vi "RT Driver VI.vi"(6 "Device Clock":string, 9 "Device Inputs FIFO":refnum<k33>, 10 "Device Outputs FIFO":refnum<k33>, 11 "Device Reference":T1 format="%.0x") -> ()   [LabVIEW 2020, in "Regatron G5 Custom Device Engine.lvlib"]
uses:
  Regatron G5 Custom Device Engine.lvlib
  <vilib>/NI VeriStand/Custom Device API/Custom Device Item Ref.ctl
  <vilib>/NI VeriStand/Custom Device API/Custom Device Channel Type.ctl
  <vilib>/Platform/TimedLoop/XDataNode/timing_clust.ctl
  <vilib>/Platform/TimedLoop/XDataNode/nitl_modes.ctl
  <vilib>/Platform/TimedLoop/XDataNode/wakeup.ctl
  G5 LabVIEW REST API/Regatron.G5.Rest Handle.llb/G5.Rest Status.ctl
  G5 LabVIEW REST API/Regatron.G5.Rest System.llb/G5.Rest System Output References Datasource.ctl
  G5 LabVIEW REST API/Regatron.G5.Rest System.llb/G5.Rest System Output Limits Datasource.ctl
  G5 LabVIEW REST API/Regatron.G5.Rest System.llb/G5.Rest System Output Limits.ctl
  G5 LabVIEW REST API/Regatron.G5.Rest System.llb/G5.Rest System Output References.ctl
  G5 LabVIEW REST API/Regatron.G5.Rest System.llb/G5.Rest System Clear Inicidents.ctl
  <userlib>/_OpenG.lib/array/array.llb/Search 1D Array (Boolean)__ogtk.vi
  <vilib>/platform/TimedLoop/XDataNode/XDataNode.xnode
  <vilib>/NI VeriStand/Custom Device API/Custom Device API.lvlib
  <vilib>/NI VeriStand/Custom Device Tools/Custom Device Utility Library/Custom Device Utility Library.lvlib
  <vilib>/Platform/TimedLoop/XDataNode/XDNodeRunTimeDep.lvlib
  G5 LabVIEW REST API/Regatron.G5.Rest.lvlib
panel:
  in  "Initialization Status Notifier":refnum<notifier>
  in  "Status Notifier":refnum<notifier>
  # "Custom Device Template\nv1.0"
  # "Use this template as a starting point for creating a custom device code module. The input controls shown here are specially named controls that the system will use to provide the device loop with data. The controls are not required for the device loop to run. For instance, if the device doesn't produce any output data, then you don't need the Device Outputs FIFO control. If you do use these controls, however, they need to have these exact names to be functional."
  # "The optional status notifier element is used to notify the RT engine of the last state of the custom device, and to indicate the device has completed execution. If this control is not used, a default No Error value is returned to the system when the device finishes execution.\n\nNote: This error state is not checked until the system shuts down. Use an output status channel to send more immediate status values to the system."
  # "This optional input can be used to send the VeriStand Engine the final status of the custom device initalization process. If this control exists on the custom device front panel, the VeriStand Engine will wait for a status update before starting up. If the custom device reports an error, that will abort the execution of the current configuration in the VeriStand Engine.\n\nThis control can be deleted if the custom device does not need to send the initialization status update."
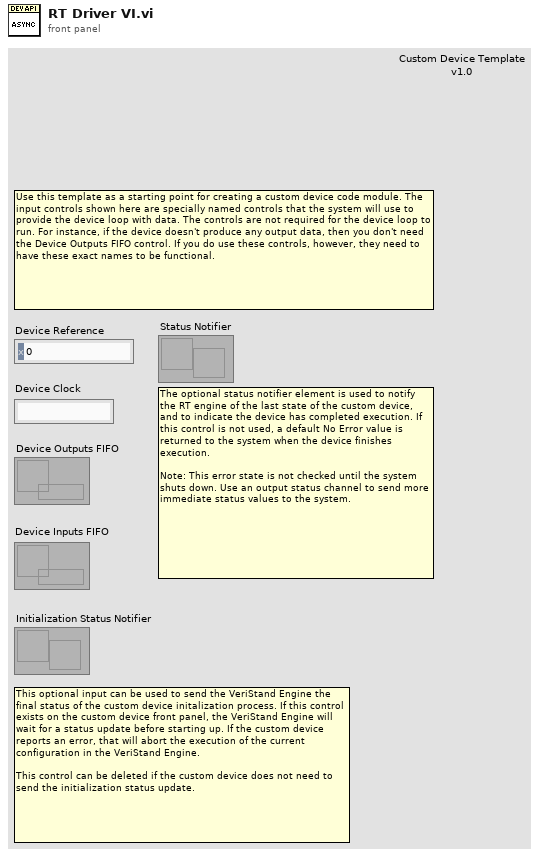
[diagram p1: front panel]
types:
  T1 = typedef "Custom Device API.lvlib/Custom Device Item Ref.ctl" = u64
  T2 = typedef "Custom Device API.lvlib/Custom Device Channel Type.ctl" = enum16{"Input", "Output"}
  T3 = typedef "XDNodeRunTimeDep.lvlib/nitl_modes.ctl" = enum32{"No Change", "Process missed periods, maintain original phase", "Discard missed periods, maintain original phase", "Process missed periods, ignore original phase", "Discard missed periods, ignore original phase"}
  T4 = typedef "XDNodeRunTimeDep.lvlib/timing_clust.ctl" = cluster{"Expected End [f-1]":u64, "Actual End [f-1]":u64, "Finished Late? [f-1]":bool, "Expected End [i-1]":u64, "Actual End [i-1]":u64, "Finished Late? [i-1]":bool, "Expected Start [i]":u64, "Actual Start [i]":u64, "Expected Start [f]":u64, "Actual Start [f]":u64, "Source Name":string, "Structure Name":string, "Period":i64, "Deadline":i64, "Offset":i64, "Start":i64, "Priority":i32, "Timeout":i32, "Mode":T3, "Wakeup Reason":T5, "Error":errorcluster, "Source Type":string, "Secondary Source Type":string, "Global End Time":u64, "Global Start Time":u64, "Frame Duration":u64, "Iteration Duration":u64, "Assigned CPU":i32, "I/O Scan Engine Mode":u32}
  T5 = typedef "XDNodeRunTimeDep.lvlib/wakeup.ctl" = enum32{"Normal", "Aborted", "Asynchronous wakeup", "Timing source error", "Timed loop error", "Timeout"}
  T6 = typedef "Regatron G5 Custom Device Shared.lvlib/Regatron.G5.Rest.lvlib/G5.Rest Status.ctl" = enum16{"Read", "Write"}
  T7 = typedef "Regatron G5 Custom Device Shared.lvlib/Regatron.G5.Rest.lvlib/G5.Rest System Output Limits.ctl" = cluster{"Voltage Upper Limit V":sgl, "Voltage Lower Limit V":sgl, "Current Upper Limit A":sgl, "Current Lower Limit A":sgl, "Power Upper Limit W":sgl, "Power Lower Limit W":sgl}
  T8 = typedef "Regatron G5 Custom Device Shared.lvlib/Regatron.G5.Rest.lvlib/G5.Rest System Output References.ctl" = cluster{"Voltage V":sgl, "Current A":sgl, "Power W":sgl, "Load R Ohm":sgl}
  T9 = typedef "Regatron G5 Custom Device Shared.lvlib/Regatron.G5.Rest.lvlib/G5.Rest System Clear Inicidents.ctl" = enum16{"Clear Errors and Warnings", "Clear Warnings", "Clear Errors"}
  T10 = typedef "Custom Device API.lvlib/Custom Device Timed Loop Priority.ctl" = enum32{"Low", "Medium", "High"}
  T11 = typedef "Regatron G5 Custom Device Shared.lvlib/Regatron.G5.Rest.lvlib/G5.Rest System Output References Datasource.ctl" = enum16{"Voltage", "Current", "Power", "Load Resistance", "ALL"}[]
  T12 = typedef "Regatron G5 Custom Device Shared.lvlib/Regatron.G5.Rest.lvlib/G5.Rest System Output Limits Datasource.ctl" = enum16{"Voltage Upper Limit", "Voltage Lower Limit", "Current Upper Limit", "Current Lower Limit", "Power Upper Limit", "Power Lower Limit", "ALL"}[]
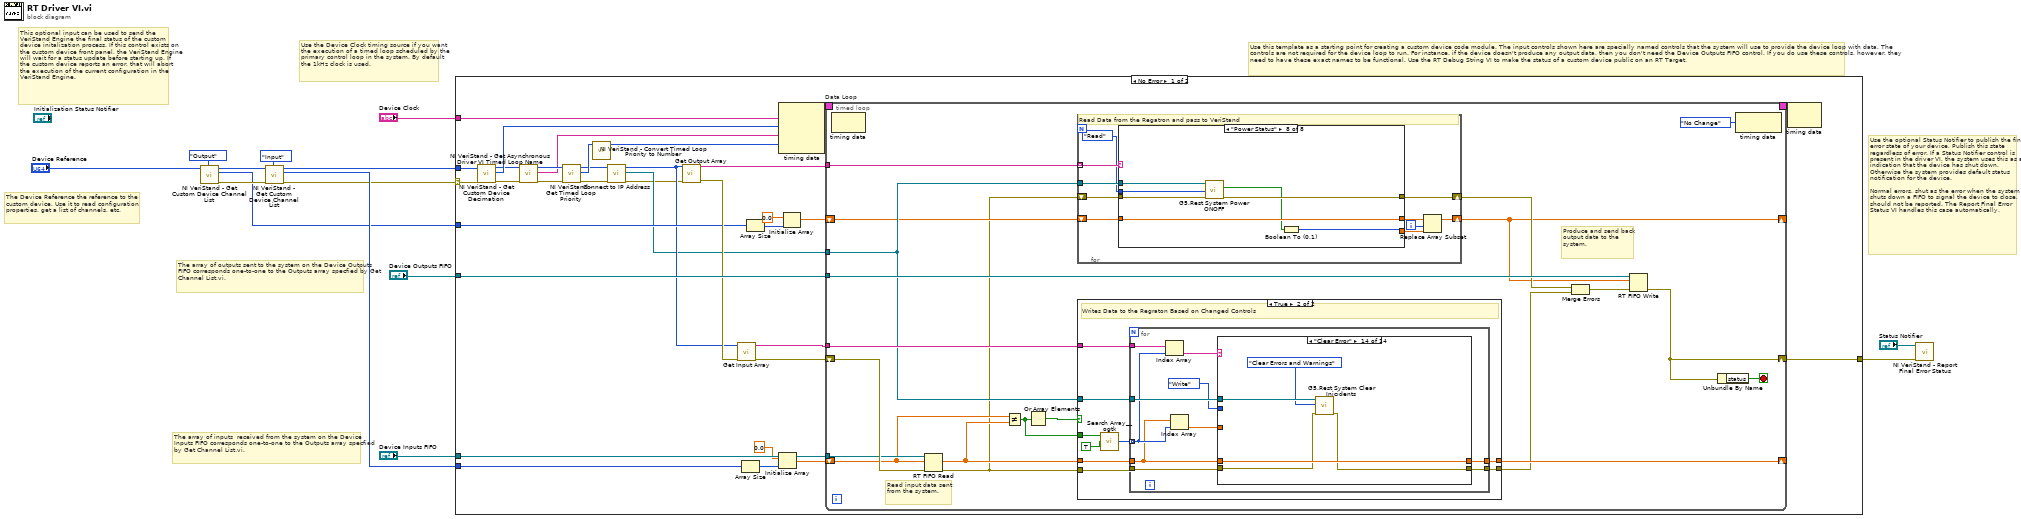
[diagram p0: block diagram]
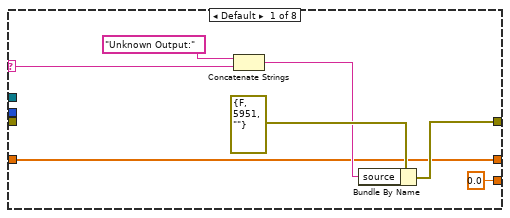
[diagram p2: hidden frame]
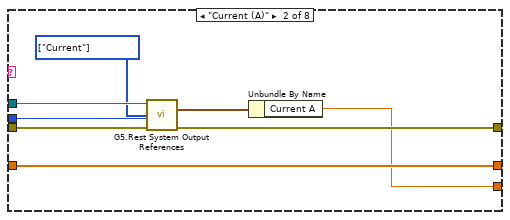
[diagram p3: hidden frame]
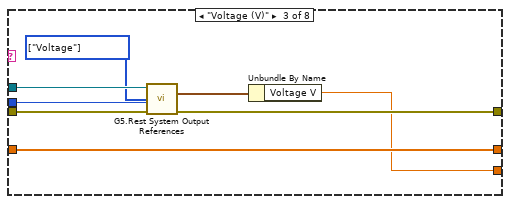
[diagram p4: hidden frame]
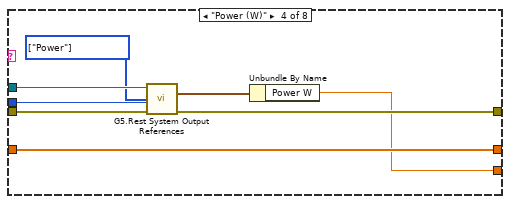
[diagram p5: hidden frame]
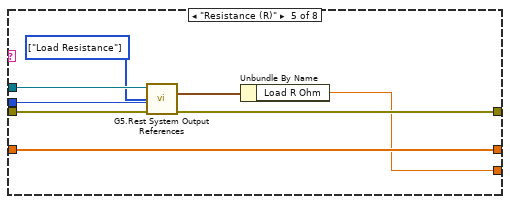
[diagram p6: hidden frame]
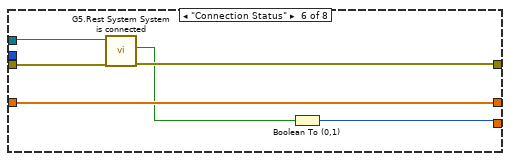
[diagram p7: hidden frame]
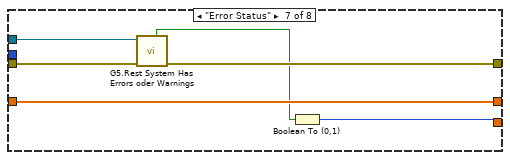
[diagram p8: hidden frame]
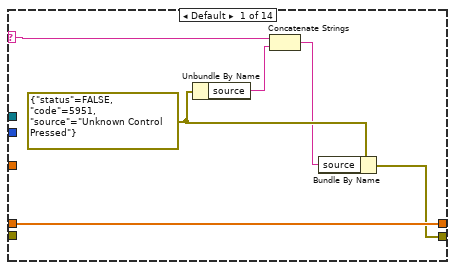
[diagram p10: hidden frame]
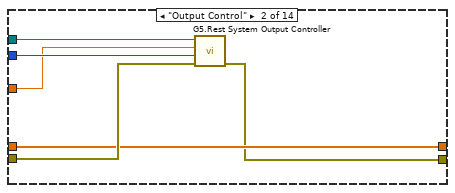
[diagram p11: hidden frame]
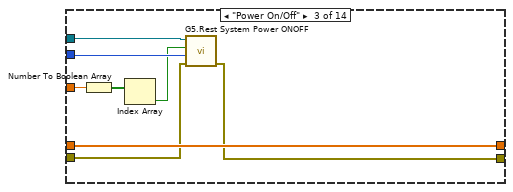
[diagram p12: hidden frame]
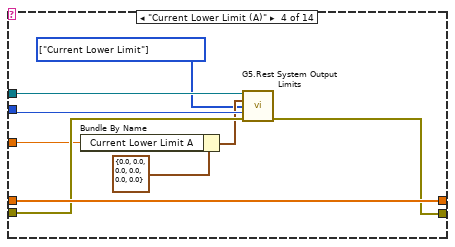
[diagram p13: hidden frame]
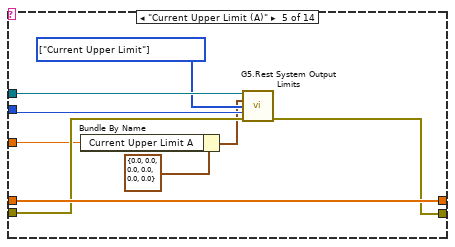
[diagram p14: hidden frame]
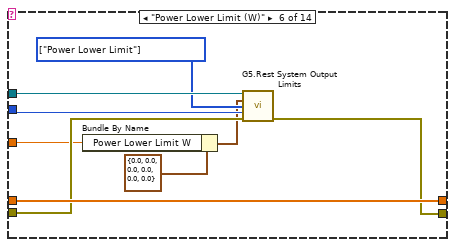
[diagram p15: hidden frame]
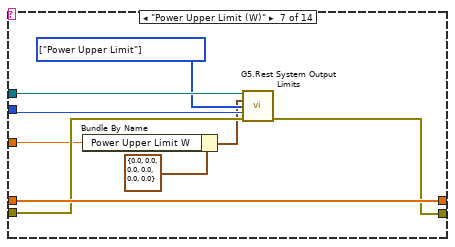
[diagram p16: hidden frame]
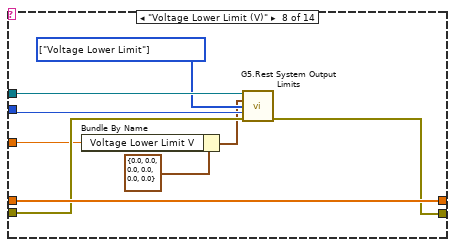
[diagram p17: hidden frame]
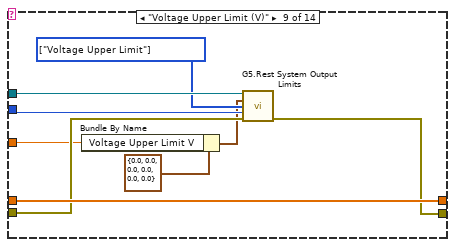
[diagram p18: hidden frame]
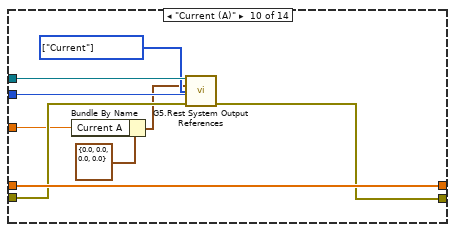
[diagram p19: hidden frame]
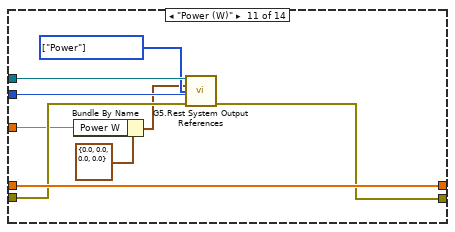
[diagram p20: hidden frame]
diagram:
  # "This optional input can be used to send the VeriStand Engine the final status of the custom device initalization process. If this control exists on the custom device front panel, the VeriStand Engine will wait for a status update before starting up. If the custom device reports an error, that will abort the execution of the current configuration in the VeriStand Engine."
  # "The array of inputs  received from the system on the Device Inputs FIFO corresponds one-to-one to the Outputs array specfied by Get Channel List.vi."
  # "Use the optional Status Notifier to publish the final error state of your device. Publish this state regardless of error. If a Status Notifier control is present in the driver VI, the system uses this as an indication that the device has shut down. Otherwise the system provides default status notification for the device.\n\nNormal errors, shut as the error when the system shuts down a FIFO to signal the device to close, should not be reported. The Report Final Error Status VI handles this case automatically."
  # "The array of outputs sent to the system on the Device Outputs FIFO corresponds one-to-one to the Outputs array specfied by Get Channel List.vi."
  # "The Device Reference the reference to the custom device. Use it to read configuration properties, get a list of channels, etc."
  # "Use the Device Clock timing source if you want the execution of a timed loop scheduled by the primary control loop in the system. By default the 1kHz clock is used."
  # "Use this template as a starting point for creating a custom device code module. The input controls shown here are specially named controls that the system will use to provide the device loop with data. The controls are not required for the device loop to run. For instance, if the device doesn't produce any output data, then you don't need the Device Outputs FIFO control. If you do use these controls, however, they need to have these exact names to be functional. Use the RT Debug String VI to make the status of a custom device public on an RT Target."
  n1 = call <vilib>:"NI VeriStand - Get Custom Device Channel List.vi"("Channel Type"=Custom_Device_Channel_Type."Output", "Device Ref in"="Device Reference") -> ("error out"=w11:errorcluster, "Specified Channel Ref List"=w2:T1[], "Device Ref out"=w5:T1)  [unwired: 1 in, 6 out]
  n2 = call <vilib>:"NI VeriStand - Get Custom Device Channel List.vi"("Channel Type"=Custom_Device_Channel_Type."Input", "error in (no error)"=w11, "Device Ref in"=w5) -> ("error out"=w3:errorcluster, "Specified Channel Ref List"=w9:T1[], "Device Ref out"=w4:T1)  [unwired: 6 out]
  n3 = case shown="No Error" w3 {
    selector: w3 -> [w31 w283]
    tunnel: "Device Outputs FIFO" -> [w47 _]
    tunnel: "Device Inputs FIFO" -> [w46 _]
    tunnel: w9 -> [w38 _]
    tunnel: [w39 w283] -> w6
    tunnel: w4 -> [w32 _]
    tunnel: w2 -> [w19 _]
    tunnel: "Device Clock" -> [w16 _]
    frame No Error {
      n4 = call <vilib>:"NI VeriStand - Get Custom Device Decimation.vi"("error in (no error)"=w31, "Device Ref in"=w32) -> ("error out"=w27:errorcluster, "Decimation"=w30:i32, "Device Ref out"=w28:T1)  [unwired: 7 in]
      n5 = call <vilib>:"NI VeriStand - Get Asynchronous Driver VI Timed Loop Name.vi"("error in (no error)"=w27, "Device Ref in"=w28) -> ("error out"=w26:errorcluster, "Device Timed Loop Name"=w24:string, "Device Ref out"=w25:T1)  [unwired: 7 in]
      n6 = call <vilib>:"NI VeriStand - Get Timed Loop Priority.vi"("error in (no error)"=w26, "Device Ref in"=w25) -> ("error out"=w20:errorcluster, "Priority"=w23:T10, "Device Ref out"=w21:T1)  [unwired: 7 in]
      n7 = call <vilib>:"NI VeriStand - Convert Timed Loop Priority to Number.vi"("Priority"=w23) -> ("Numeric Priority"=w22:i32)  [unwired: 10 in]
      n8 = call "Connect to IP Address.vi"("error in (no error)"=w20, "Device Ref in"=w21) -> ("error out"=w15:errorcluster, "REST Client out"=w17:refnum<class "REST Client.lvclass">, "Item Ref out"=w18:T1)  [unwired: 7 in]
      n9 = call "Get Output Array.vi"("error in"=w15, "Device Ref in"=w18) -> ("error out"=w29:errorcluster, "Array"=w35:string[])  [unwired: 8 in]
      n10 = call "Get Input Array.vi"("error in"=w29, "Device Ref in"=w18) -> ("error out"=w36:errorcluster, "Array"=w37:string[])  [unwired: 8 in]
      n11 = Array Size(array=w38) -> (size(s)=w40:i32)
      n12 = Array Size(array=w19) -> (size(s)=w41:i32)
      n13 = node-c288(w16, w30, w24, w22) -> (w34:T4)
      n14 = Initialize Array(0.0 ("element"), w40) -> (w42:dbl[])
      n15 = Initialize Array(0.0 ("element"), w41) -> (w43:dbl[])
      n16 = timed-loop "Data Loop" {
        shift-right: [w66] -> _
        shift-left: w42 -> [w62]
        shift-right: [w63] -> w39
        shift-left: w36 -> [w67]
        shift-right: [w50] -> _
        shift-left: w43 -> [w52]
        tunnel: w47 -> [w65]
        tunnel: w46 -> [w64]
        tunnel: w17 -> [w55]
        tunnel: w37 -> [w61]
        tunnel: w35 -> [w56]
        timing: w34 -> [_]
        timing-out: [_] -> w33
        stop <- w49 stop-if-true
        # "Produce and send back output data to the system."
        # "Read input data sent from the system."
        n17 = node-c288() -> ()  [unwired: 1 in, 1 out]
        n18 = RT FIFO Read(0:w64, 1:w62, 3:w67) -> (9:w58:dbl[], 11:w51:errorcluster)  [unwired: 4 out]
        n19 = Not Equal?(x=w62, y=w58) -> (x != y?=w60:bool[])
        n20 = Or Array Elements(Boolean array=w60) -> (logical OR=w57:bool)
        n21 = for {
          tunnel: w56 -> [w81] mode=indexing
          tunnel: w55 -> [w80]
          shift-right: [w79] -> w53
          shift-left: w51 -> [w77]
          shift-right: [w73] -> w50
          shift-left: w52 -> [w78]
          i -> [w75]
          # "Read Data from the Regatron and pass to VeriStand"
          n22 = case shown="\"Power Status\"" w81 {
            selector: w81 -> [w83 _ _ _ _ _ _ _]
            tunnel: w80 -> [_ w96 w104 w112 w120 w125 w130 w136]
            tunnel: w77 -> [_ w95 w103 w111 w119 w124 w129 w137]
            tunnel: G5.Rest_Status."Read" ("Status") -> [_ w94 w102 w110 w118 _ _ w133]
            tunnel: [w86 w93 w101 w109 w117 w123 w128 w135] -> w79
            tunnel: w78 -> [w84 w92 w100 w108 w116 w126 w132 w139]
            tunnel: [w84 w92 w100 w108 w116 w126 w132 w139] -> w76
            tunnel: [sgl 0.0 ("Load R Ohm") w90 w98 w106 w114 w121 w131 w138] -> w74
            frame Default {
              n23 = Concatenate Strings("Unknown Output:" ("string"), w83) -> (w87:string)
              n24 = Bundle By Name(cluster=errorcluster {"status"=FALSE, "code"=5951, "source"=""} ("Fehler (Ausgang)"), "source"=w87) -> (w86:errorcluster)
            }
            frame "Current (A)" {
              w89 = T11 [enum."Current"] items=["Voltage", "Current", "Power", "Load Resistance", "ALL"] ("Datasource")
              n25 = call "G5.Rest System Output References .vi"("G5 WEB API (Eingang)"=w96, "Datasource"=w89, "Status"=w94, "Fehler (Eingang, kein Fehler)"=w95) -> ("GET Output Reference"=w91:T8, "Fehler (Ausgang)"=w93:errorcluster)  [unwired: 9 in, 1 out]
              n26 = Unbundle By Name(w91) -> ("Current A"=w90:sgl)
            }
            frame "Voltage (V)" {
              w97 = T11 [enum."Voltage"] items=["Voltage", "Current", "Power", "Load Resistance", "ALL"] ("Datasource")
              n27 = call "G5.Rest System Output References .vi"("G5 WEB API (Eingang)"=w104, "Datasource"=w97, "Status"=w102, "Fehler (Eingang, kein Fehler)"=w103) -> ("GET Output Reference"=w99:T8, "Fehler (Ausgang)"=w101:errorcluster)  [unwired: 9 in, 1 out]
              n28 = Unbundle By Name(w99) -> ("Voltage V"=w98:sgl)
            }
            frame "Power (W)" {
              w105 = T11 [enum."Power"] items=["Voltage", "Current", "Power", "Load Resistance", "ALL"] ("Datasource")
              n29 = call "G5.Rest System Output References .vi"("G5 WEB API (Eingang)"=w112, "Datasource"=w105, "Status"=w110, "Fehler (Eingang, kein Fehler)"=w111) -> ("GET Output Reference"=w107:T8, "Fehler (Ausgang)"=w109:errorcluster)  [unwired: 9 in, 1 out]
              n30 = Unbundle By Name(w107) -> ("Power W"=w106:sgl)
            }
            frame "Resistance (R)" {
              w113 = T11 [enum."Load Resistance"] items=["Voltage", "Current", "Power", "Load Resistance", "ALL"] ("Datasource")
              n31 = call "G5.Rest System Output References .vi"("G5 WEB API (Eingang)"=w120, "Datasource"=w113, "Status"=w118, "Fehler (Eingang, kein Fehler)"=w119) -> ("GET Output Reference"=w115:T8, "Fehler (Ausgang)"=w117:errorcluster)  [unwired: 9 in, 1 out]
              n32 = Unbundle By Name(w115) -> ("Load R Ohm"=w114:sgl)
            }
            frame "Connection Status" {
              n33 = call "G5.Rest System System is connected.vi"("Fehler (Eingang, kein Fehler)"=w124, "G5 WEB API (Eingang)"=w125) -> ("Fehler (Ausgang)"=w123:errorcluster, "System is connected"=w122:bool)  [unwired: 7 in, 1 out]
              n34 = Boolean To (0,1)(Boolean=w122) -> (0, 1=w121:i16)
            }
            frame "Error Status" {
              n35 = call "G5.Rest System Has Errors oder Warnings.vi"("Fehler (Eingang, kein Fehler)"=w129, "G5 WEB API (Eingang)"=w130) -> ("Fehler (Ausgang)"=w128:errorcluster, "System has Errors or Warnings"=w127:bool)  [unwired: 5 in, 3 out]
              n36 = Boolean To (0,1)(Boolean=w127) -> (0, 1=w131:i16)
            }
            frame "Power Status" {
              n37 = call "G5.Rest System Power ONOFF.vi"("Fehler (Eingang, kein Fehler)"=w137, "Status"=w133, "G5 WEB API (Eingang)"=w136) -> ("Fehler (Ausgang)"=w135:errorcluster, "Get Power OFF/ON"=w134:bool)  [unwired: 6 in, 1 out]
              n38 = Boolean To (0,1)(Boolean=w134) -> (0, 1=w138:i16)
            }
          }
          n39 = Replace Array Subset(array=w76, new element=w74, index=w75) -> (w73:dbl[])
        }
        n40 = case shown="True" w57 {
          tunnel: w55 -> [_ w150]
          tunnel: w51 -> [w141 w149]
          tunnel: w60 -> [_ w148]
          tunnel: w61 -> [_ w145]
          tunnel: [w141 w144] -> w59
          tunnel: w58 -> [w140 w143]
          tunnel: [w140 w142] -> w66
          frame False {
          }
          frame True {
            # "Writes Data to the Regraton Based on Changed Controls"
            n41 = call-poly <userlib>:"Search Array__ogtk.vi"("Array"=w148, "Element Data"=TRUE) -> ("Indices of Elements"=w146:i32[])  [unwired: 7 in]
            n42 = for {
              tunnel: w150 -> [w160]
              tunnel: w149 -> [w159]
              tunnel: w146 -> [w156] mode=indexing
              tunnel: w145 -> [w158]
              tunnel: [w154] -> w144
              tunnel: w143 -> [w153]
              tunnel: [w152] -> w142
              n43 = Index Array(array=w158, index=w156) -> (element=w157:string)
              n44 = Index Array(array=w153, index=w156) -> (element=w155:dbl)
              n45 = case shown="\"Clear Error\"" w157 {
                selector: w157 -> [w162 _ _ _ _ _ _ _ _ _ _ _ _ _]
                tunnel: w160 -> [_ w172 w179 w188 w197 w206 w215 w224 w233 w242 w251 w260 w269 w274]
                tunnel: G5.Rest_Status."Write" ("Status") -> [_ w171 w178 w187 w196 w205 w214 w223 w232 w241 w250 w259 w268 _]
                tunnel: w159 -> [_ w170 w177 w186 w195 w204 w213 w222 w231 w240 w249 w258 w267 w273]
                tunnel: w155 -> [_ w169 w174 w183 w193 w202 w211 w220 w229 w239 w248 w257 w266 _]
                tunnel: [w164 w167 w173 w185 w194 w203 w212 w221 w230 w238 w247 w256 w265 w272] -> w154
                tunnel: w153 -> [w166 w168 w180 w189 w198 w207 w216 w225 w234 w243 w252 w261 w270 w275]
                tunnel: [w166 w168 w180 w189 w198 w207 w216 w225 w234 w243 w252 w261 w270 w275] -> w152
                frame Default {
                  w165 = errorcluster {"status"=FALSE, "code"=5951, "source"="Unknown Control Pressed"} ("Fehler (Ausgang)")
                  n46 = Unbundle By Name(w165) -> ("source"=w163:string)
                  n47 = Concatenate Strings(w162, w163) -> (w161:string)
                  n48 = Bundle By Name(cluster=w165, "source"=w161) -> (w164:errorcluster)
                }
                frame "Output Control" {
                  n49 = call "G5.Rest System Output Controller.vi"("Fehler (Eingang, kein Fehler)"=w170, "Status"=w171, "SET Output Control"=w169, "G5 WEB API (Eingang)"=w172) -> ("Fehler (Ausgang)"=w167:errorcluster)  [unwired: 5 in, 2 out]
                }
                frame "Power On/Off" {
                  n50 = Number To Boolean Array(number=w174) -> (Boolean array=w176:bool[])
                  n51 = Index Array(array=w176) -> (element=w175:bool)  [unwired: 1 in]
                  n52 = call "G5.Rest System Power ONOFF.vi"("Fehler (Eingang, kein Fehler)"=w177, "Status"=w178, "Power OFF/ON"=w175, "G5 WEB API (Eingang)"=w179) -> ("Fehler (Ausgang)"=w173:errorcluster)  [unwired: 5 in, 2 out]
                }
                frame "Current Lower Limit (A)" {
                  w182 = T12 [enum."Current Lower Limit"] items=["Voltage Upper Limit", "Voltage Lower Limit", "Current Upper Limit", "Current Lower Limit", "Power Upper Limit", "Power Lower Limit", "ALL"] ("Datasource")
                  n53 = Bundle By Name(cluster=T7 {"Voltage Upper Limit V"=0.0, "Voltage Lower Limit V"=0.0, "Current Upper Limit A"=0.0, "Current Lower Limit A"=0.0, "Power Upper Limit W"=0.0, "Power Lower Limit W"=0.0} ("SET Output Limit"), "Current Lower Limit A"=w183) -> (w184:T7)
                  n54 = call "G5.Rest System Output Limits.vi"("G5 WEB API (Eingang)"=w188, "SET Output Limit"=w184, "Datasource"=w182, "Status"=w187, "Fehler (Eingang, kein Fehler)"=w186) -> ("Fehler (Ausgang)"=w185:errorcluster)  [unwired: 8 in, 2 out]
                }
                frame "Current Upper Limit (A)" {
                  w192 = T12 [enum."Current Upper Limit"] items=["Voltage Upper Limit", "Voltage Lower Limit", "Current Upper Limit", "Current Lower Limit", "Power Upper Limit", "Power Lower Limit", "ALL"] ("Datasource")
                  n55 = Bundle By Name(cluster=T7 {"Voltage Upper Limit V"=0.0, "Voltage Lower Limit V"=0.0, "Current Upper Limit A"=0.0, "Current Lower Limit A"=0.0, "Power Upper Limit W"=0.0, "Power Lower Limit W"=0.0} ("SET Output Limit"), "Current Upper Limit A"=w193) -> (w190:T7)
                  n56 = call "G5.Rest System Output Limits.vi"("G5 WEB API (Eingang)"=w197, "SET Output Limit"=w190, "Datasource"=w192, "Status"=w196, "Fehler (Eingang, kein Fehler)"=w195) -> ("Fehler (Ausgang)"=w194:errorcluster)  [unwired: 8 in, 2 out]
                }
                frame "Power Lower Limit (W)" {
                  w201 = T12 [enum."Power Lower Limit"] items=["Voltage Upper Limit", "Voltage Lower Limit", "Current Upper Limit", "Current Lower Limit", "Power Upper Limit", "Power Lower Limit", "ALL"] ("Datasource")
                  n57 = Bundle By Name(cluster=T7 {"Voltage Upper Limit V"=0.0, "Voltage Lower Limit V"=0.0, "Current Upper Limit A"=0.0, "Current Lower Limit A"=0.0, "Power Upper Limit W"=0.0, "Power Lower Limit W"=0.0} ("SET Output Limit"), "Power Lower Limit W"=w202) -> (w199:T7)
                  n58 = call "G5.Rest System Output Limits.vi"("G5 WEB API (Eingang)"=w206, "SET Output Limit"=w199, "Datasource"=w201, "Status"=w205, "Fehler (Eingang, kein Fehler)"=w204) -> ("Fehler (Ausgang)"=w203:errorcluster)  [unwired: 8 in, 2 out]
                }
                frame "Power Upper Limit (W)" {
                  w210 = T12 [enum."Power Upper Limit"] items=["Voltage Upper Limit", "Voltage Lower Limit", "Current Upper Limit", "Current Lower Limit", "Power Upper Limit", "Power Lower Limit", "ALL"] ("Datasource")
                  n59 = Bundle By Name(cluster=T7 {"Voltage Upper Limit V"=0.0, "Voltage Lower Limit V"=0.0, "Current Upper Limit A"=0.0, "Current Lower Limit A"=0.0, "Power Upper Limit W"=0.0, "Power Lower Limit W"=0.0} ("SET Output Limit"), "Power Upper Limit W"=w211) -> (w208:T7)
                  n60 = call "G5.Rest System Output Limits.vi"("G5 WEB API (Eingang)"=w215, "SET Output Limit"=w208, "Datasource"=w210, "Status"=w214, "Fehler (Eingang, kein Fehler)"=w213) -> ("Fehler (Ausgang)"=w212:errorcluster)  [unwired: 8 in, 2 out]
                }
                frame "Voltage Lower Limit (V)" {
                  w219 = T12 [enum."Voltage Lower Limit"] items=["Voltage Upper Limit", "Voltage Lower Limit", "Current Upper Limit", "Current Lower Limit", "Power Upper Limit", "Power Lower Limit", "ALL"] ("Datasource")
                  n61 = Bundle By Name(cluster=T7 {"Voltage Upper Limit V"=0.0, "Voltage Lower Limit V"=0.0, "Current Upper Limit A"=0.0, "Current Lower Limit A"=0.0, "Power Upper Limit W"=0.0, "Power Lower Limit W"=0.0} ("SET Output Limit"), "Voltage Lower Limit V"=w220) -> (w217:T7)
                  n62 = call "G5.Rest System Output Limits.vi"("G5 WEB API (Eingang)"=w224, "SET Output Limit"=w217, "Datasource"=w219, "Status"=w223, "Fehler (Eingang, kein Fehler)"=w222) -> ("Fehler (Ausgang)"=w221:errorcluster)  [unwired: 8 in, 2 out]
                }
                frame "Voltage Upper Limit (V)" {
                  w228 = T12 [enum."Voltage Upper Limit"] items=["Voltage Upper Limit", "Voltage Lower Limit", "Current Upper Limit", "Current Lower Limit", "Power Upper Limit", "Power Lower Limit", "ALL"] ("Datasource")
                  n63 = Bundle By Name(cluster=T7 {"Voltage Upper Limit V"=0.0, "Voltage Lower Limit V"=0.0, "Current Upper Limit A"=0.0, "Current Lower Limit A"=0.0, "Power Upper Limit W"=0.0, "Power Lower Limit W"=0.0} ("SET Output Limit"), "Voltage Upper Limit V"=w229) -> (w226:T7)
                  n64 = call "G5.Rest System Output Limits.vi"("G5 WEB API (Eingang)"=w233, "SET Output Limit"=w226, "Datasource"=w228, "Status"=w232, "Fehler (Eingang, kein Fehler)"=w231) -> ("Fehler (Ausgang)"=w230:errorcluster)  [unwired: 8 in, 2 out]
                }
                frame "Current (A)" {
                  w237 = T11 [enum."Current"] items=["Voltage", "Current", "Power", "Load Resistance", "ALL"] ("Datasource")
                  n65 = Bundle By Name(cluster=T8 {"Voltage V"=0.0, "Current A"=0.0, "Power W"=0.0, "Load R Ohm"=0.0} ("SET Output Reference"), "Current A"=w239) -> (w235:T8)
                  n66 = call "G5.Rest System Output References .vi"("G5 WEB API (Eingang)"=w242, "SET Output Reference"=w235, "Datasource"=w237, "Status"=w241, "Fehler (Eingang, kein Fehler)"=w240) -> ("Fehler (Ausgang)"=w238:errorcluster)  [unwired: 8 in, 2 out]
                }
                frame "Power (W)" {
                  w246 = T11 [enum."Power"] items=["Voltage", "Current", "Power", "Load Resistance", "ALL"] ("Datasource")
                  n67 = Bundle By Name(cluster=T8 {"Voltage V"=0.0, "Current A"=0.0, "Power W"=0.0, "Load R Ohm"=0.0} ("SET Output Reference"), "Power W"=w248) -> (w244:T8)
                  n68 = call "G5.Rest System Output References .vi"("G5 WEB API (Eingang)"=w251, "SET Output Reference"=w244, "Datasource"=w246, "Status"=w250, "Fehler (Eingang, kein Fehler)"=w249) -> ("Fehler (Ausgang)"=w247:errorcluster)  [unwired: 8 in, 2 out]
                }
                frame "Resistance (R)" {
                  w255 = T11 [enum."Load Resistance"] items=["Voltage", "Current", "Power", "Load Resistance", "ALL"] ("Datasource")
                  n69 = Bundle By Name(cluster=T8 {"Voltage V"=0.0, "Current A"=0.0, "Power W"=0.0, "Load R Ohm"=0.0} ("SET Output Reference"), "Load R Ohm"=w257) -> (w253:T8)
                  n70 = call "G5.Rest System Output References .vi"("G5 WEB API (Eingang)"=w260, "SET Output Reference"=w253, "Datasource"=w255, "Status"=w259, "Fehler (Eingang, kein Fehler)"=w258) -> ("Fehler (Ausgang)"=w256:errorcluster)  [unwired: 8 in, 2 out]
                }
                frame "Voltage (V)" {
                  w264 = T11 [enum."Voltage"] items=["Voltage", "Current", "Power", "Load Resistance", "ALL"] ("Datasource")
                  n71 = Bundle By Name(cluster=T8 {"Voltage V"=0.0, "Current A"=0.0, "Power W"=0.0, "Load R Ohm"=0.0} ("SET Output Reference"), "Voltage V"=w266) -> (w262:T8)
                  n72 = call "G5.Rest System Output References .vi"("G5 WEB API (Eingang)"=w269, "SET Output Reference"=w262, "Datasource"=w264, "Status"=w268, "Fehler (Eingang, kein Fehler)"=w267) -> ("Fehler (Ausgang)"=w265:errorcluster)  [unwired: 8 in, 2 out]
                }
                frame "Clear Error" {
                  n73 = call "G5.Rest System Clear Inicidents.vi"("Fehler (Eingang, kein Fehler)"=w273, "Clear Inicidents"=G5.Rest_System_Clear_Inicidents."Clear Errors and Warnings", "G5 WEB API (Eingang)"=w274) -> ("Fehler (Ausgang)"=w272:errorcluster)  [unwired: 7 in, 1 out]
                }
              }
            }
          }
        }
        n74 = Merge Errors(w53, w59) -> (w54:errorcluster)
        n75 = RT FIFO Write(0:w65, 1:w50, 3:w54) -> (11:w63:errorcluster)  [unwired: 1 in, 4 out]
        n76 = Unbundle By Name(w63) -> ("status"=w49:bool)
        n77 = node-c288(nitl_modes."No Change" ("Mode")) -> ()  [unwired: 1 out]
      }
      n78 = node-c288(w33) -> ()  [unwired: 1 out]
    }
    frame Error {
    }
  }
  n79 = call <vilib>:"NI VeriStand - Report Final Error Status.vi"("error in (no error)"=w6, "Status Notifier"="Status Notifier") -> ()  [unwired: 1 in, 9 out]
